vi "Get Trigger Model State.vi"(8 "error in (no error)":errorcluster, 11 "VISA resource name":refnum<visa-resource-name>) -> (0 "error out":errorcluster, 1 "Block Number":string, 2 "Trigger Mode State":string, 3 "VISA resource name out":refnum<visa-resource-name>)   [LabVIEW 2015, in "Keithley 2450.lvlib"]
doc: "This Vi returns the present state of the trigger model."
uses:
  <instrlib>/Keithley 2450/Keithley 2450.lvlib
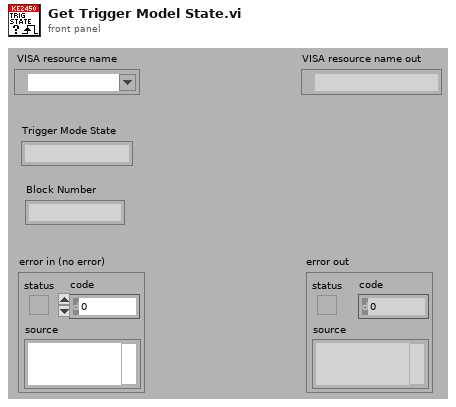
[diagram p1: front panel]
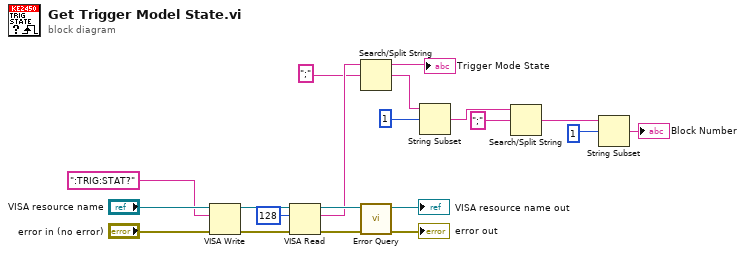
[diagram p0: block diagram]
diagram:
  n1 = VISA Write(VISA resource name="VISA resource name", write buffer=":TRIG:STAT?" ("format string"), error in (no error)="error in (no error)") -> (VISA resource name out=w14:refnum<visa-resource-name>, error out=w16:errorcluster)  [unwired: 1 out]
  n2 = VISA Read(VISA resource name=w14, byte count=u32 128, error in (no error)=w16) -> (VISA resource name out=w13:refnum<visa-resource-name>, read buffer=w9:string, error out=w15:errorcluster)  [unwired: 1 out]
  n3 = Search/Split String(string=w9, search string/char (-)=";") -> (substring before match=→"Trigger Mode State":string, match + rest of string=w7:string)  [unwired: 1 in, 1 out]
  n4 = call <instrlib>:"Error Query.vi"("error in (no error)"=w15, "VISA resource name"=w13) -> ("error out"=→"error out":errorcluster, "VISA resource name out"=→"VISA resource name out":refnum<visa-resource-name>)  [unwired: 8 out]
  n5 = String Subset(string=w7, offset (0)=1) -> (substring=w4:string)  [unwired: 1 in]
  n6 = Search/Split String(string=w4, search string/char (-)=";") -> (match + rest of string=w3:string)  [unwired: 1 in, 2 out]
  n7 = String Subset(string=w3, offset (0)=1) -> (substring=→"Block Number":string)  [unwired: 1 in]
